vi "Process.vi"(8 "error in":errorcluster, 11 "system":refnum<class "system.lvclass">) -> (0 "error out":errorcluster, 3 "system out":refnum<class "system.lvclass">)   [LabVIEW 2016, in "system.lvclass"]
doc: "---------------------------------------------------------------\nJKI State Machine Objects™\nhttp://jki.net/state-machine-objects/\nCopyright (C) 2005-2015, JKI <info@jki.net>\nALL RIGHTS RESERVED"
uses:
  system.lvclass
  <vilib>/JKI/JKI SMO/SMO/SMO.lvclass
  <vilib>/JKI/JKI SMO/SMO/Typedefs/Parent Call--Enum.ctl
  instrument/instrument.lvclass
  DAQ_Manager/DAQ_Manager.lvclass
  DSP/DSP.lvclass
  C:/user/patrick/hg/levy_inst_lockin.SMO/lvsrc/SMOs/instrument/instrument.lvclass
  C:/Program Files (x86)/National Instruments/LabVIEW 2016/vi.lib/JKI/JKI SMO/SMO/SMO.lvclass
  Generator/Generator.lvclass
  DAQmx.AO/Typedefs/DAQmx.AO_Config.ctl
  DAQmx.AO/DAQmx.AO.lvclass
  DAQ/Typedefs/DAQ_Config.ctl
  DAQ/DAQ.lvclass
  DAQ/Typedefs/DAQ_SamplingMode.ctl
  DAQ/Typedefs/DAQ_SamplingInfo.ctl
  DAQ/Typedefs/PrivateEvents--DAQ.AI.Channels.ctl
  DAQ/Typedefs/DAQ_Type.ctl
  DAQmx.AI/Typedefs/DAQmx.AI_Config.ctl
  DAQmx.AI/DAQmx.AI.lvclass
  DAQmx.AI/Typedefs/AI.Coupling-enum.ctl
  DAQmx.AI/Typedefs/AI.Terminal-enum.ctl
  DAQmx.AO/Typedefs/AO.Terminal-enum.ctl
  DSP/Typedefs/LP_Config.ctl
  DSP.lockin/Typedefs/Lockin_Config.ctl
  DSP.lockin/DSP_lockin.lvclass
  <vilib>/Analysis/4window.llb/windowTd.ctl
  <vilib>/Analysis/NI_AALPro.lvlib
  <vilib>/measure/maspectr.llb/Power Spectrum and PSD Export Mode.ctl
  <vilib>/measure/NI_MAPro.lvlib
  DSP/Typedefs/FFT_Config.ctl
  DSP/Typedefs/PrivateEvents--DSP.RunCalculation.ctl
panel:
  in  "Tab Control":enum32{"process FP", "DAQ", "AO", "DSP"}(tab)
  in  "Simulate?":bool
  out "str":string
  in  "show UI?":bool
  in  "DAQmx Physical Channels (AI)":tag="PXI1Slot2/ai0:1, PXI1Slot3/ai0:1, PXI1Slot4/ai0:1, PXI1Slot5/ai0:1, PXI1Slot6/ai0:1, PXI1Slot7/ai0:1"
  in  "DAQmx.AO.config":T1={"output terminal configuration"=-1} {"output terminal configuration" items=["Default"=-1, "RSE"=10083, "Differential"=10106, "Pseudodifferential"=12529]}
  in  "DAQmx Physical Channels (AO)":tag="PXI1Slot2/ao0:1, PXI1Slot3/ao0:1, PXI1Slot4/ao0:1, PXI1Slot5/ao0:1, PXI1Slot6/ao0:1, PXI1Slot7/ao0:1"
  in  "DAQ.Config (AO)":T3={"Channels"="", "DAQ_Type"=enum."AO", "minimum value"=-10.0, "maximum value"=10.0, "DAQ_SamplingInfo"={"Fs"=1000.0, "#s"=1000}, "DAQ_SamplingMode"=enum."Continuous"} {"maximum value" format="%0.2f"; "minimum value" format="%0.2f"}
  in  "DAQ.Config (AI)":T3={"Channels"="", "DAQ_Type"=enum."AI", "minimum value"=-10.0, "maximum value"=10.0, "DAQ_SamplingInfo"={"Fs"=1000.0, "#s"=1000}, "DAQ_SamplingMode"=enum."Continuous"} {"maximum value" format="%0.2f"; "minimum value" format="%0.2f"}
  in  "DAQmx.AI.config":T8={"AI.Coupling"=10045, "input terminal configuration "=-1} {"input terminal configuration" items=["default"=-1, "RSE"=10083, "NRSE"=10078, "Differential"=10106, "Pseudodifferential"=12529]; "AI.Coupling" items=["AC"=10045, "DC"=10050, "GND"=10066]}
  in  "runCalculation":T11={"runCalculation"={"adjust gain"=FALSE, "subtract offset"=FALSE, "60 Hz prefilter"=FALSE, "LP prefilter"=FALSE, "lockin"=FALSE, "FFT"=FALSE, "gain"=[], "offset"=[], "LP config"={"high cutoff freq [Hz]"=0.45}, "Lockin config"=[], "FFT config"={"averaging parameters"={"averaging mode"=enum."RMS averaging", "weighting mode"=enum."Exponential", "number of averages"=10}, "window"=1, "export mode"=0, "window parameter"=nan, "restart averaging (F)"=FALSE}}} {"runCalculation"."FFT config"."export mode" items=["Power Spectrum", "Power Spectral Density"]; "runCalculation"."FFT config"."window" items=["Rectangle"=0, "Hanning"=1, "Hamming"=2, "Blackman-Harris"=3, "Exact Blackman"=4, "Blackman"=5, "Flat Top"=6, "4 Term B-Harris "=7, "7 Term B-Harris"=8, "Low Sidelobe"=9, "Blackman Nuttall"=11, "Triangle"=30, "Bartlett-Hanning"=31, "Bohman"=32, "Parzen"=33, "Welch"=34, "Kaiser"=60, "Dolph-Chebyshev"=61, "Gaussian"=62]; "runCalculation"."FFT config"."averaging parameters"."number of averages" min=1; "runCalculation"."Lockin config"."TC (s)" format="%#_13g"}
  # "system process.vi"
  # "For instructions on how to use the JKI State Machine Objects, examples and video tutorials, visit:\nhttp://jki.net/state-machine-objects/\n\nJKI State Machine Objects™\nhttp://jki.net/state-machine-objects/\nCopyright (C) 2005-2015, JKI <info@jki.net>\nALL RIGHTS RESERVED"
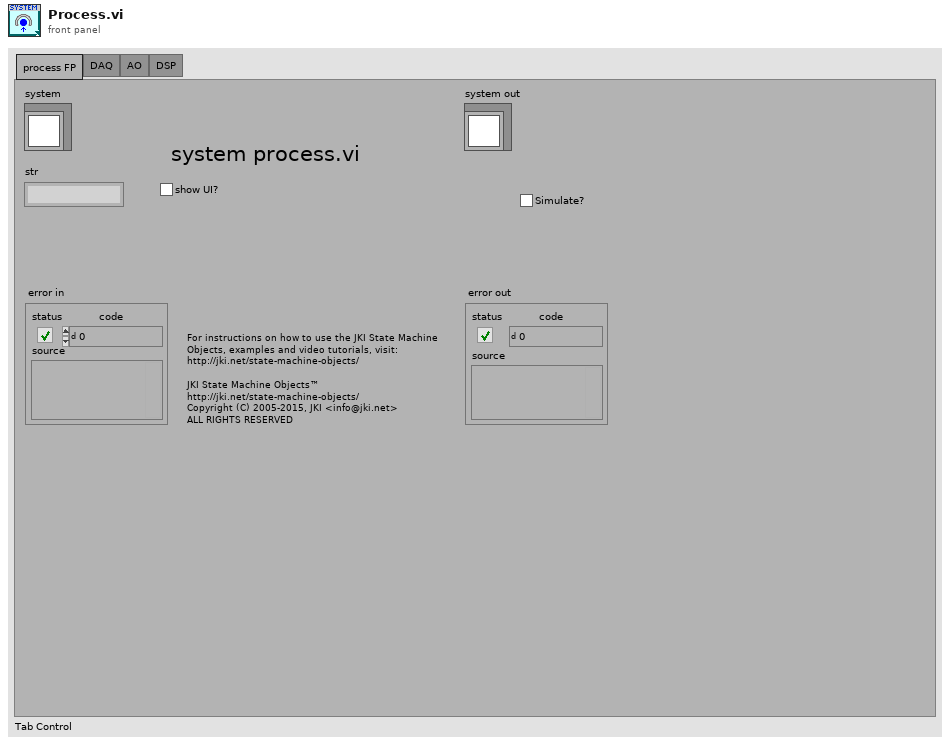
[diagram p1: front panel]
types:
  T1 = typedef "DAQmx.AO.lvclass/DAQmx.AO_Config.ctl" = cluster{"output terminal configuration":T2}
  T2 = typedef "DAQmx.AO.lvclass/AO.Terminal-enum.ctl" = i32
  T3 = typedef "DAQ.lvclass/DAQ_Config.ctl" = cluster{"Channels":T4, "DAQ_Type":T5, "minimum value":dbl, "maximum value":dbl, "DAQ_SamplingInfo":T6, "DAQ_SamplingMode":T7}
  T4 = typedef "DAQ.lvclass/PrivateEvents--DAQ.AI.Channels.ctl" = string
  T5 = typedef "DAQ.lvclass/DAQ_Type.ctl" = enum16{"AI", "AO"}
  T6 = typedef "DAQ.lvclass/DAQ_SamplingInfo.ctl" = cluster{"Fs":dbl, "#s":i32}
  T7 = typedef "DAQ.lvclass/DAQ_SamplingMode.ctl" = enum16{"Continuous", "Finite"}
  T8 = typedef "DAQmx.AI.lvclass/DAQmx.AI_Config.ctl" = cluster{"AI.Coupling":T9, "input terminal configuration ":T10}
  T9 = typedef "DAQmx.AI.lvclass/AI.Coupling-enum.ctl" = i32
  T10 = typedef "DAQmx.AI.lvclass/AI.Terminal-enum.ctl" = i32
  T11 = typedef "DSP.lvclass/PrivateEvents--DSP.RunCalculation.ctl" = cluster{"runCalculation":cluster{"adjust gain":bool, "subtract offset":bool, "60 Hz prefilter":bool, "LP prefilter":bool, "lockin":bool, "FFT":bool, "gain":dbl[], "offset":dbl[], "LP config":T12, "Lockin config":T13, "FFT config":T14}}
  T12 = typedef "DSP.lvclass/LP_Config.ctl" = cluster{"high cutoff freq [Hz]":dbl}
  T13 = typedef "DSP_lockin.lvclass/Lockin_Config.ctl" = cluster{" f (Hz)":dbl, "phi (deg)":dbl, "TC (s)":dbl, "order":i32}[]
  T14 = typedef "DSP.lvclass/FFT_Config.ctl" = cluster{"averaging parameters":cluster{"averaging mode":enum16{"No averaging", "Vector averaging", "RMS averaging", "Peak hold"}, "weighting mode":enum16{"Linear", "Exponential"}, "number of averages":u32}, "window":T15, "export mode":T16, "window parameter":dbl, "restart averaging (F)":bool}
  T15 = typedef "NI_AALPro.lvlib/windowTd.ctl" = u32
  T16 = typedef "NI_MAPro.lvlib/Power Spectrum and PSD Export Mode.ctl" = u16
  T17 = typedef "SMO.lvclass/Parent Call--Enum.ctl" = enum16{"Allows parent to run", "Does not request parent to run"}
  T18 = enum32{"invalid app kind", "Development System", "Run Time System", "Student Edition", "Embedded LabVIEW", "Evaluation", "Custom"}
  T19 = enum32{"Invalid", "Standard", "Closed", "Hidden", "Minimized", "Maximized"}
  T20 = enum32{"Bad", "Idle", "Run top level", "Running"}
  T21 = typedef "DAQ_Manager.lvclass/PublicEvents--DAQ_Manager.getWaveform.ctl" = waveform(dbl)[]
  T22 = cluster{"Core":cluster{"Current VI Reference":refnum<vi>, "Close Panel on Exit?":bool, "error":errorcluster}, "Self Reference":refnum<class "system.lvclass">, "Your string data":string, "to":i32, "AI Array":waveform(dbl)[], "AO Array":waveform(dbl)[], "DAQ_Manager":refnum<class "DAQ_Manager.lvclass">, "DSP":refnum<class "DSP.lvclass">, "Generator":refnum<class "Generator.lvclass">, "Scope":refnum<class "Scope.lvclass">}
  T23 = typedef "Generator.lvclass/PublicEvents--Generator.getGeneratorWaveforms.ctl" = waveform(dbl)[]
  T24 = cluster{"Current VI Reference":refnum<vi>, "Close Panel on Exit?":bool, "error":errorcluster}
  T25 = typedef "SMO.lvclass/Protected Events.ctl" = cluster{"StopProcesses":refnum<user-event>, "AbortProcesses":refnum<user-event>, "Config Changed":refnum<user-event>, "Dependency":refnum<user-event>}
  T26 = typedef "system.lvclass/PrivateEvents--Cluster.ctl" = cluster{"output_config":refnum<user-event>, "lockin_config":refnum<user-event>, "lockin_REF_waveform":refnum<user-event>}
  T27 = cluster{"SMO Protected Events":T25, "Private Events":T26}
  T28 = typedef "SMO.lvclass/Public Events.ctl" = cluster{"Error":refnum<user-event>, "State":refnum<user-event>, "Reserve State":refnum<user-event>}
  T29 = typedef "DAQ_Manager.lvclass/PublicEvents--Cluster.ctl" = cluster{"getWaveform":refnum<user-event>}
  T30 = cluster{"Public Events":T28, "Public Events":T29}
  T31 = typedef "DSP.lvclass/PublicEvents--Cluster.ctl" = cluster{"getWaveforms":refnum<user-event>, "getLockin":refnum<user-event>, "getPowerSpectrum":refnum<user-event>}
  T32 = cluster{"Public Events":T28, "Public Events":T31}
  T33 = typedef "Generator.lvclass/PublicEvents--Cluster.ctl" = cluster{"getGeneratorWaveforms":refnum<user-event>}
  T34 = cluster{"Public Events":T28, "Public Events":T33}
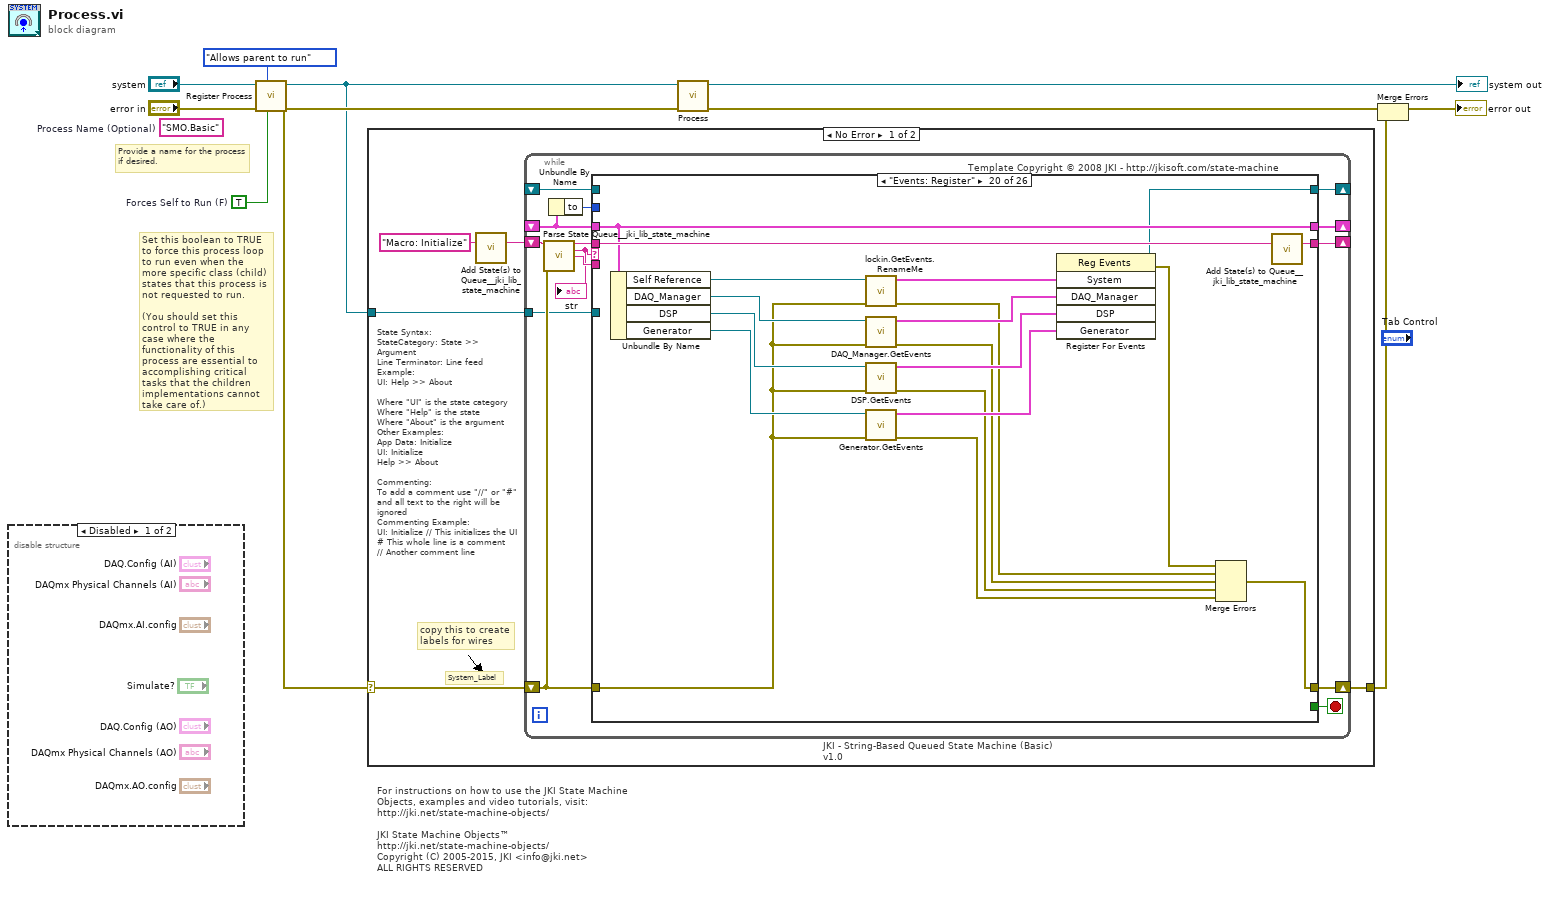
[diagram p0: block diagram]
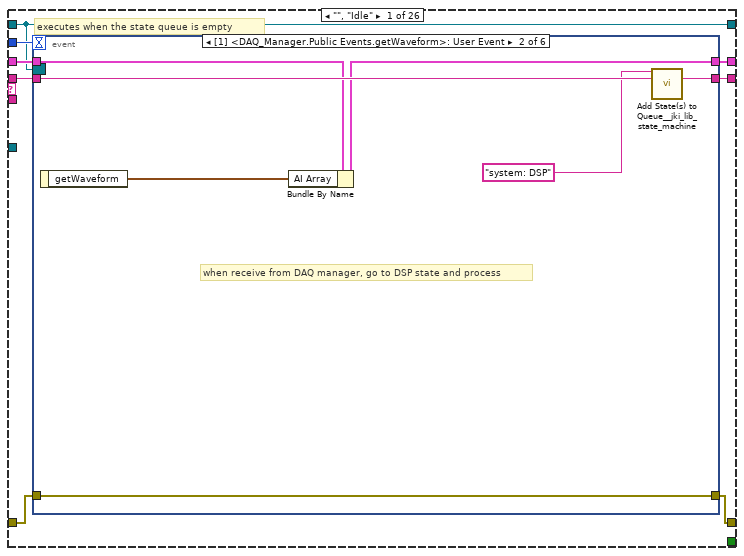
[diagram p3: hidden frame]
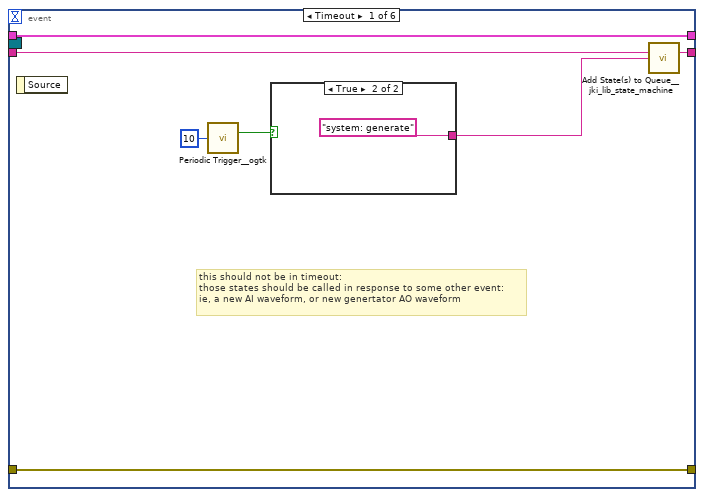
[diagram p4: hidden frame]
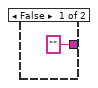
[diagram p5: hidden frame]
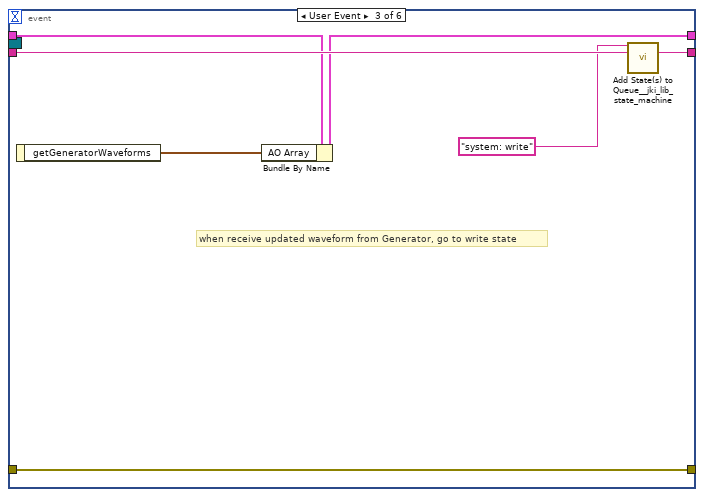
[diagram p6: hidden frame]
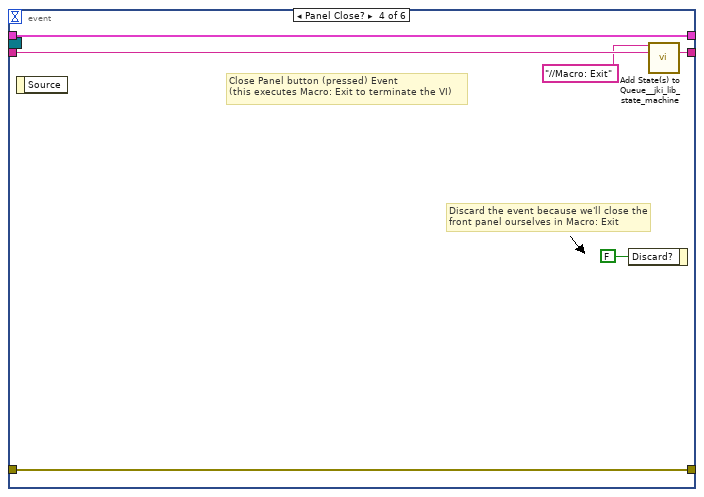
[diagram p7: hidden frame]
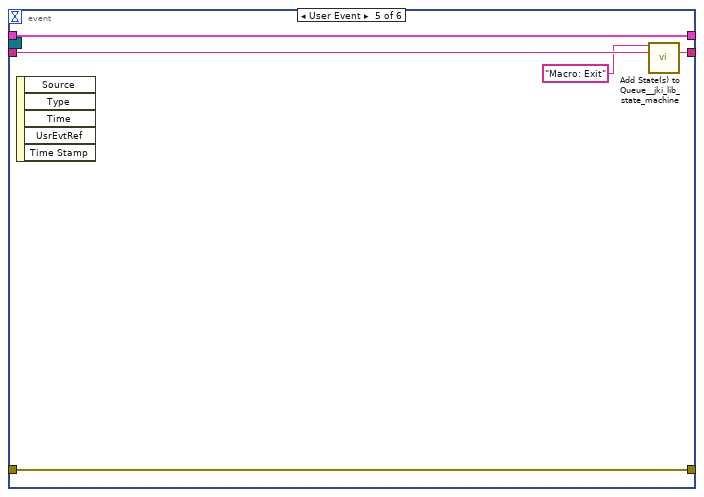
[diagram p8: hidden frame]
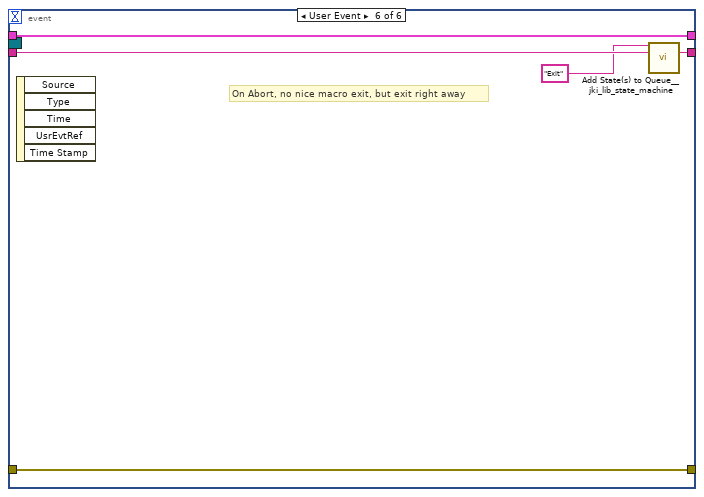
[diagram p9: hidden frame]
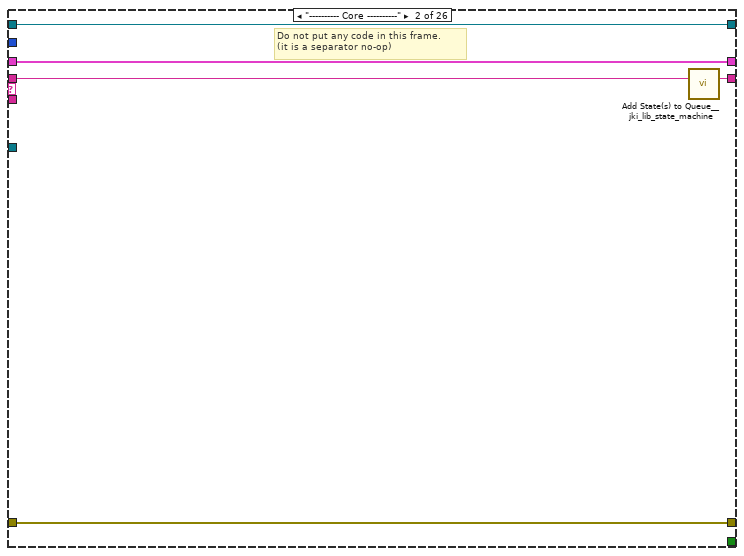
[diagram p10: hidden frame]
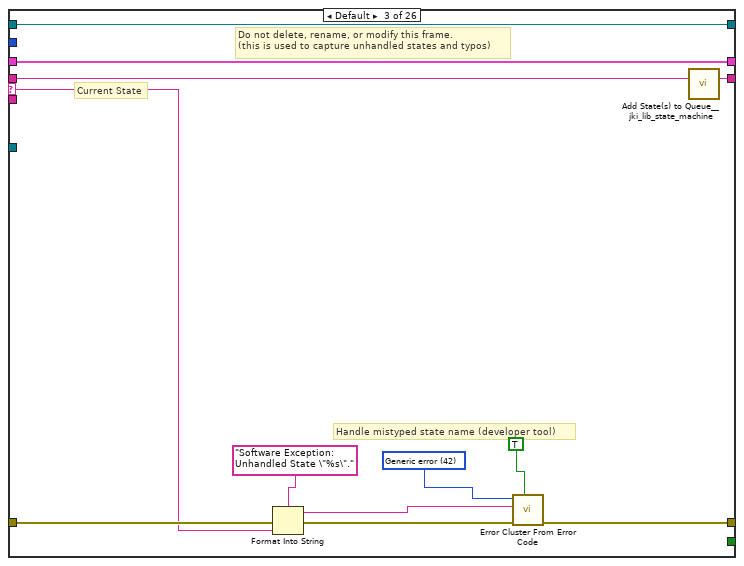
[diagram p11: hidden frame]
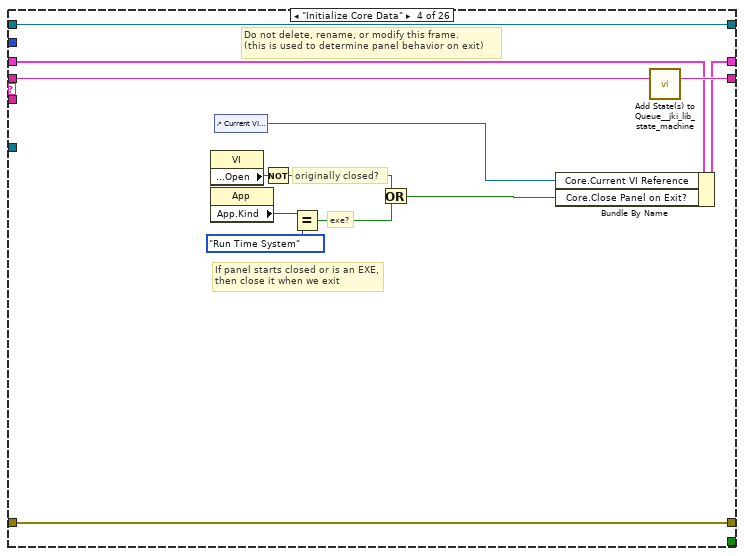
[diagram p12: hidden frame]
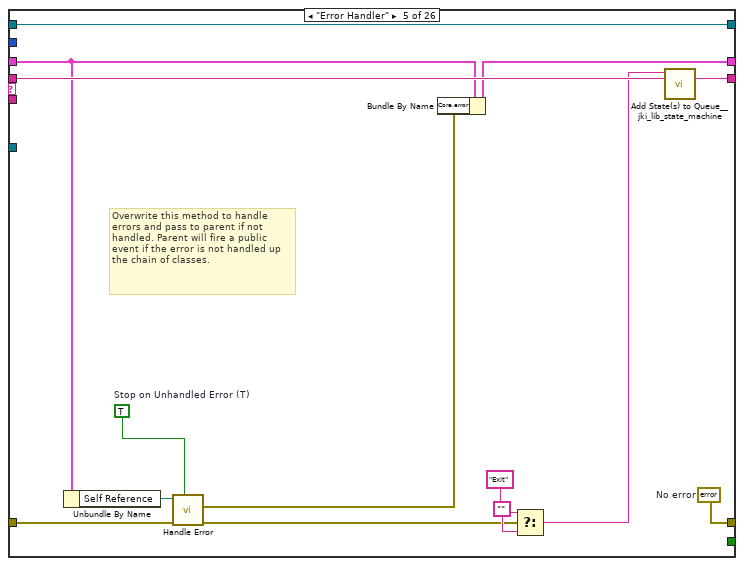
[diagram p13: hidden frame]
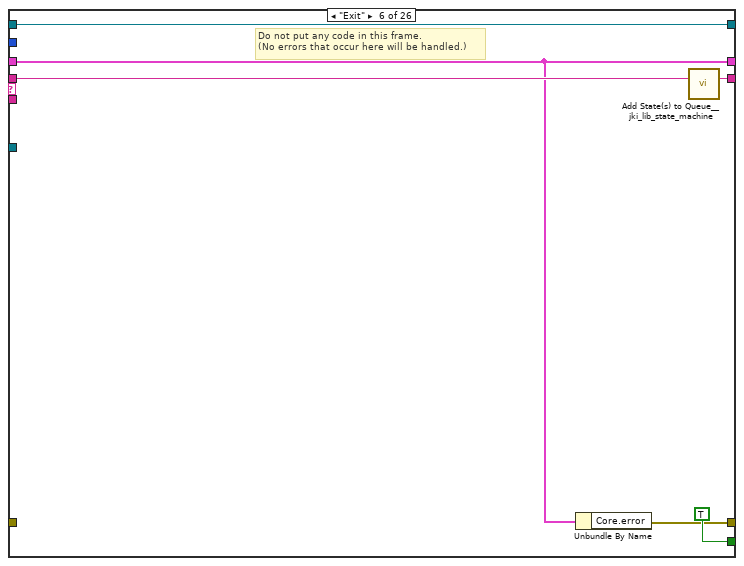
[diagram p14: hidden frame]
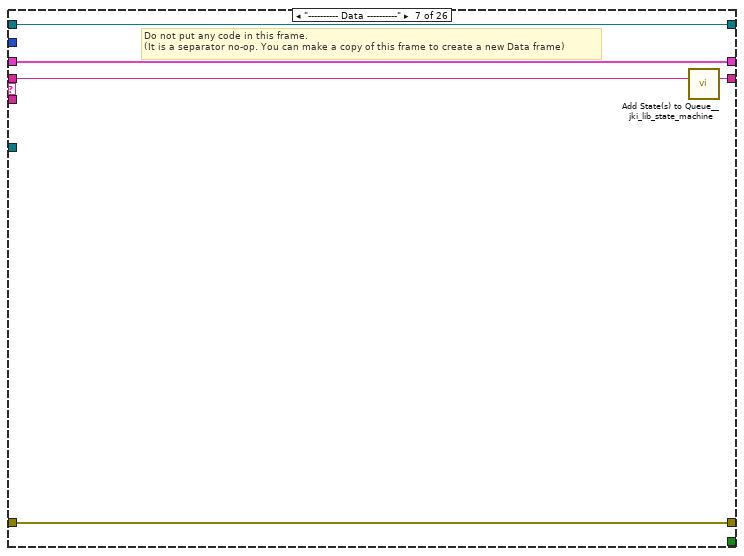
[diagram p15: hidden frame]
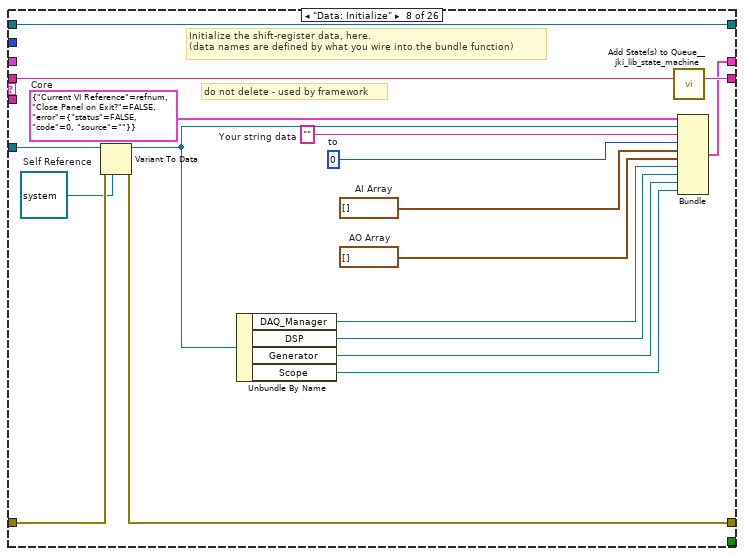
[diagram p16: hidden frame]
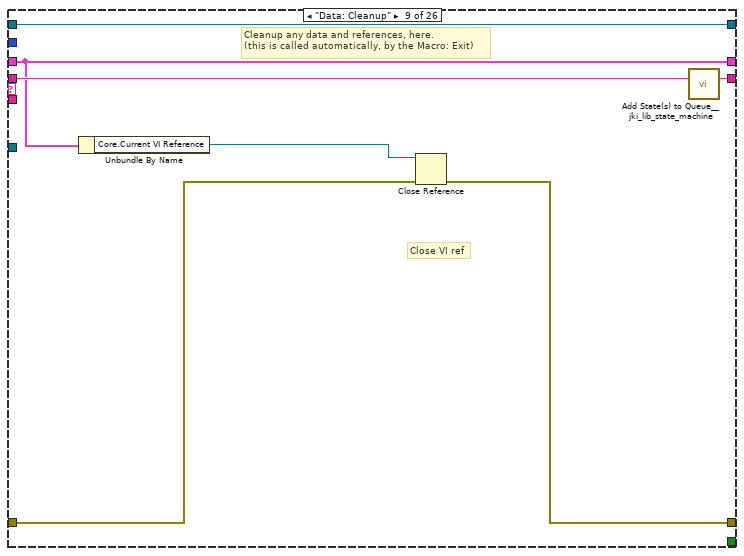
[diagram p17: hidden frame]
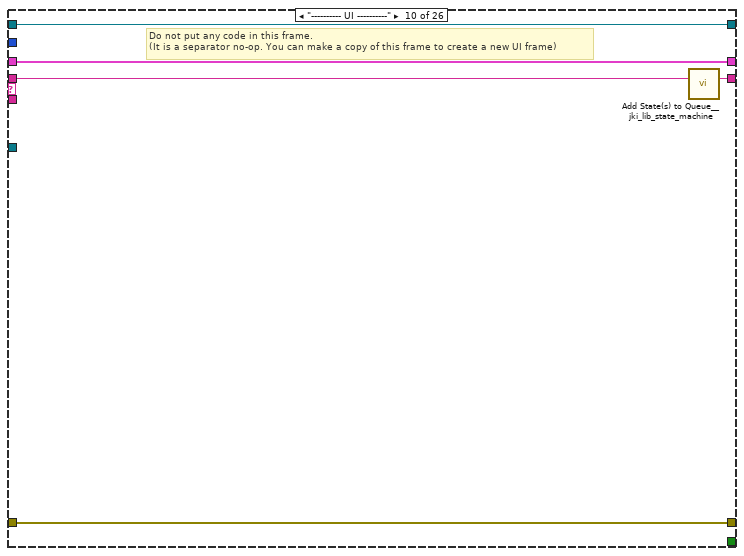
[diagram p18: hidden frame]
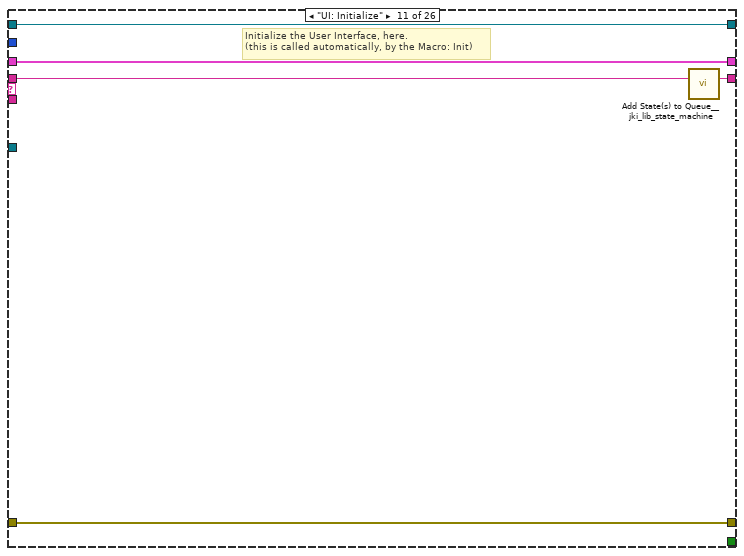
[diagram p19: hidden frame]
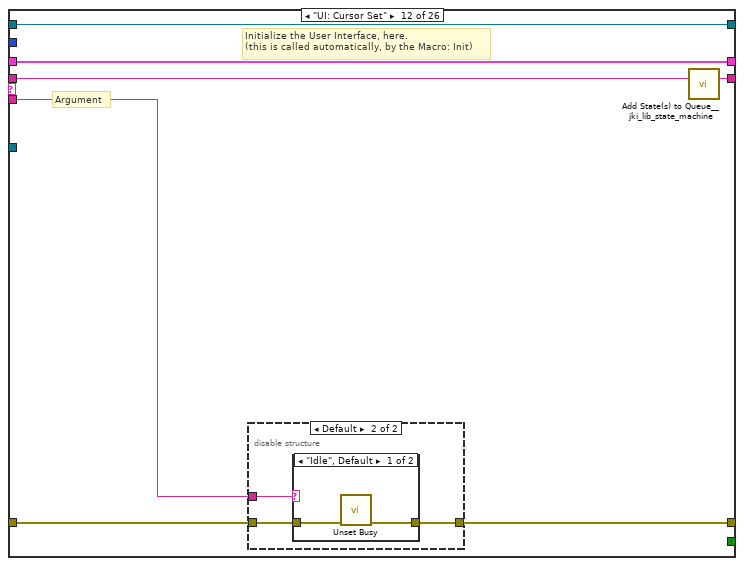
[diagram p20: hidden frame]
diagram:
  w1 = TRUE  # Forces Self to Run (F)
  (unwired) "SMO.Basic"  # Process Name (Optional)
  # "Provide a name for the process\nif desired."
  # "Set this boolean to TRUE to force this process loop to run even when the more specific class (child) states that this process is not requested to run.\n\n(You should set this control to TRUE in any case where the functionality of this process are essential to accomplishing critical tasks that the children implementations cannot take care of.)"
  # "For instructions on how to use the JKI State Machine Objects, examples and video tutorials, visit:\nhttp://jki.net/state-machine-objects/\n\nJKI State Machine Objects™\nhttp://jki.net/state-machine-objects/\nCopyright (C) 2005-2015, JKI <info@jki.net>\nALL RIGHTS RESERVED"
  n1 = disable-structure shown="Disabled" {
    frame Disabled {
    }
    frame Enabled {
    }
  }
  n2 = call <vilib>:"Register Process.vi"("Forces Self to Run (F)"=w1, "Parent Call"=Parent_Call--Enum."Allows parent to run", "error in (no error)"="error in", "SMO"="system") -> ("error out"=w7:errorcluster, "SMO out"=w6:refnum<class "system.lvclass">)  [unwired: 6 in]
  n3 = case shown="No Error" w7 {
    selector: w7 -> [w12 w346]
    tunnel: w6 -> [w13 _]
    tunnel: [w11 w346] -> w3
    frame No Error {
      # "State Syntax:\nStateCategory: State >> Argument\nLine Terminator: Line feed\nExample:\nUI: Help >> About\n\nWhere \"UI\" is the state category\nWhere \"Help\" is the state\nWhere \"About\" is the argument\nOther Examples:\nApp Data: Initialize\nUI: Initialize\nHelp >> About\n\nCommenting:\nTo add a comment use \"//\" or \"#\" and all text to the right will be ignored\nCommenting Example:\nUI: Initialize // This initializes the UI\n# This whole line is a comment\n// Another comment line"
      # "copy this to create labels for wires"
      # "System_Label"
      n4 = call <vilib>:"Add State(s) to Queue__jki_lib_state_machine.vi"("State(s) in (\"\")"="Macro: Initialize") -> ("States Out"=w15:string)  [unwired: 14 in]
      n5 = while "JKI - String-Based Queued State Machine (Basic) v1.0" {
        shift-right: [w23] -> _
        shift-left: _ -> [w17]
        shift-right: [w26] -> w11
        shift-left: w12 -> [w22]
        shift-right: [w25] -> _
        shift-left: w15 -> [w27]
        tunnel: w13 -> [w21]
        shift-right: [w20] -> _
        shift-left: _ -> [w19]
        stop <- w24 stop-if-true
        # "Template Copyright © 2008 JKI - http://jkisoft.com/state-machine"
        n6 = call <vilib>:"Parse State Queue__jki_lib_state_machine.vi"("State Queue"=w27, "Error In (no error)"=w22) -> ("Remaining States"=w29:string, "Current State"=w18:string, "Arguments"=w28:string)  [unwired: 11 in]
        "str" <- w18
        n7 = Unbundle By Name(w17) -> ("to"=w16:i32)
        n8 = case shown="\"Events: Register\"" w18 {
          selector: w18 -> [_ _ w83 _ _ _ _ _ _ _ _ _ _ _ _ _ _ _ _ _ _ _ _ _ _ _]
          tunnel: w29 -> [w37 w81 w87 w106 w120 w126 w131 w149 w156 w161 w166 w173 w189 w221 w241 w255 w260 w271 w276 w295 w301 w306 w313 w325 w335 w345]
          tunnel: w28 -> [_ _ _ _ _ _ _ _ _ _ _ w167 w183 _ _ _ _ _ _ _ _ _ _ _ _ _]
          tunnel: w17 -> [w35 w78 w85 w97 w114 w122 w128 _ w152 w158 w164 w171 w185 w218 w237 w246 w257 w268 w273 w293 w299 w304 w310 w321 w331 w342]
          tunnel: [w34 w79 w89 w103 w115 w121 w129 w144 w153 w159 w163 w168 w186 w219 w239 w253 w258 w262 w274 w278 w297 w302 w307 w317 w330 w341] -> w26
          tunnel: w22 -> [w33 w79 w88 w103 w116 _ w129 w145 w151 w159 w163 w169 w187 w219 w239 w253 w258 w263 w274 w284 w297 w302 w307 w319 w330 w337]
          tunnel: [w36 w80 w86 w105 w119 w125 w130 w148 w155 w160 w165 w172 w188 w220 w240 w254 w259 w270 w275 w294 w300 w305 w312 w324 w334 w344] -> w25
          tunnel: [_ _ _ _ _ TRUE _ _ _ _ _ _ _ _ _ _ _ _ _ _ _ _ _ _ _ _] -> w24
          tunnel: [w32 w78 w85 w104 w113 w122 w128 w147 w152 w158 w164 w171 w185 w218 w237 w246 w257 w268 w273 w293 w299 w304 w309 w321 w331 w342] -> w23
          tunnel: w16 -> [w31 _ _ _ _ _ _ _ _ _ _ _ _ _ _ _ _ _ _ _ _ _ _ _ _ _]
          tunnel: w21 -> [_ _ _ _ _ _ _ w142 _ _ _ _ _ _ _ _ _ _ _ _ _ _ _ _ _ _]
          tunnel: [w30 w77 w82 w94 w118 w123 w127 w141 w154 w157 w162 w170 w182 w217 w238 w247 w256 w269 w272 w287 w298 w303 w311 w323 w333 w343] -> w20
          tunnel: w19 -> [w30 w77 w82 w94 w118 w123 w127 w141 w154 w157 w162 w170 w182 w217 w238 w247 w256 w269 w272 _ w298 w303 w311 w323 w333 w343]
          frame "", "Idle" {
            # "executes when the state queue is empty"
            n9 = event shown="[1] <DAQ_Manager.Public Events.getWaveform>: User Event" {
              selector: w30 -> [_ _ _ _ _ _]
              dyn-events: _ -> [_ _ _ _ _ _]
              timeout: w31 -> [_ _ _ _ _ _]
              tunnel: w37 -> [w44 w52 w59 w66 w71 w76]
              tunnel: [w43 w53 w60 w65 w70 w75] -> w36
              tunnel: w35 -> [w42 w50 w57 w63 w68 w73]
              tunnel: [w41 w51 w58 w64 w69 w74] -> w34
              tunnel: w33 -> [w41 w51 w58 w64 w69 w74]
              tunnel: [w42 w49 w56 w63 w68 w73] -> w32
              event Timeout {
                # "this should not be in timeout:\nthose states should be called in response to some other event:\nie, a new AI waveform, or new genertator AO waveform"
                n10 = event-data() -> ()  [unwired: 1 in, 1 out]
                n11 = call <userlib>:"Periodic Trigger__ogtk.vi"("time (ms)"=u32 10) -> ("Triggered"=w38:bool)  [unwired: 12 in, 2 out]
                n12 = case shown="True" w38 {
                  tunnel: ["" ("State(s) in Front (\"\")") "system: generate" ("State(s) in Front (\"\")")] -> w40
                  frame False {
                  }
                  frame True {
                  }
                }
                n13 = call <vilib>:"Add State(s) to Queue__jki_lib_state_machine.vi"("State(s) in (\"\")"=w44, "State(s) at Back (\"\")"=w40) -> ("States Out"=w43:string)  [unwired: 13 in]
              }
              event User Event {
                # "when receive from DAQ manager, go to DSP state and process"
                n14 = event-data() -> ("getWaveform"=w48:T21)  [unwired: 1 in]
                n15 = Bundle By Name(cluster=w50, "AI Array"=w48) -> (w49:T22)
                n16 = call <vilib>:"Add State(s) to Queue__jki_lib_state_machine.vi"("State(s) in Front (\"\")"="system: DSP" ("State(s) in Front (\"\")"), "State(s) in (\"\")"=w52) -> ("States Out"=w53:string)  [unwired: 13 in]
              }
              event User Event {
                # "when receive updated waveform from Generator, go to write state"
                n17 = event-data() -> ("getGeneratorWaveforms"=w55:T23)  [unwired: 1 in]
                n18 = Bundle By Name(cluster=w57, "AO Array"=w55) -> (w56:T22)
                n19 = call <vilib>:"Add State(s) to Queue__jki_lib_state_machine.vi"("State(s) in Front (\"\")"="system: write" ("State(s) in Front (\"\")"), "State(s) in (\"\")"=w59) -> ("States Out"=w60:string)  [unwired: 13 in]
              }
              event Panel Close? {
                # "Discard the event because we'll close the front panel ourselves in Macro: Exit"
                # "Close Panel button (pressed) Event\n(this executes Macro: Exit to terminate the VI)"
                n20 = event-data() -> ()  [unwired: 1 in, 1 out]
                n21 = event-data("Discard?"=FALSE) -> ()  [unwired: 1 in, 1 out]
                n22 = call <vilib>:"Add State(s) to Queue__jki_lib_state_machine.vi"("State(s) in Front (\"\")"="//Macro: Exit", "State(s) in (\"\")"=w66) -> ("States Out"=w65:string)  [unwired: 13 in]
              }
              event User Event {
                n23 = event-data() -> ()  [unwired: 1 in, 5 out]
                n24 = call <vilib>:"Add State(s) to Queue__jki_lib_state_machine.vi"("State(s) in Front (\"\")"="Macro: Exit", "State(s) in (\"\")"=w71) -> ("States Out"=w70:string)  [unwired: 13 in]
              }
              event User Event {
                # "On Abort, no nice macro exit, but exit right away"
                n25 = event-data() -> ()  [unwired: 1 in, 5 out]
                n26 = call <vilib>:"Add State(s) to Queue__jki_lib_state_machine.vi"("State(s) in Front (\"\")"="Exit", "State(s) in (\"\")"=w76) -> ("States Out"=w75:string)  [unwired: 13 in]
              }
            }
          }
          frame "---------- Core ----------" {
            # "Do not put any code in this frame.\n(it is a separator no-op)"
            n27 = call <vilib>:"Add State(s) to Queue__jki_lib_state_machine.vi"("State(s) in (\"\")"=w81) -> ("States Out"=w80:string)  [unwired: 14 in]
          }
          frame Default {
            w92 = 42 items=["No error", "Argument error", "Memory is full", "Out of zone", "End of file", "File already open", "Generic file I/O error", "File not found", "File permission error", "Disk is full", "Duplicate path", "Too many files open", "System feature not enabled", "Resource file not found", "Cannot add resource", "Resource not found", "Image not found", "Image memory error", "Pen does not exist", "Config type invalid", "Config token not found", "Config parse error", "Config memory error", "Bad external code format", "Bad external code offset", "External code not present", "Null window", "Destroy window error", "Null menu", "Print aborted", "Bad print record", "Print driver error", "Windows error during printing", "Memory error during printing", "Print dialog error", "Generic print error", "Invalid device refnum", "Device not found", "Device parameter error", "Device unit error", "Cannot open device", "Device call aborted", "Generic error", "Cancelled by user", "Object ID too low", "Object ID too high", "Object not in heap", "Unknown heap", "Unknown object (invalid DefProc)", "Unknown object (DefProc not in table)", "Message out of range", "Invalid (null) method", "Unknown message", "Manager call not supported", "Bad address", "Network operation in progress", "Network operation timed out", "Connection is busy", "Network attribute not supported", "Network error", "Address in use", "System out of memory", "Connection aborted", "Connection refused", "Not connected", "Already connected", "Connection closed", "Initialization error (interapplication manager)", "Bad occurrence", "Wait on unbound occurrence handler", "Occurrence queue overflow", "Datalog type conflict", "Unused", "Unrecognized type (interapplication manager)", "Memory corrupt", "Failed to make temporary DLL", "Old CIN version", "Drag socket not found", "Failed to load drop-object", "Failed to register OLE object", "Failed to release OLE object", "Format specifier type mismatch", "Unknown format specifier", "Too few format specifiers", "Too many format specifiers", "Scan failed", "Newer CIN version", "Error converting to variant", "Runtime menu error", "Password tampered", "Variant attribute not found", "Incompatible variant data type", "Event data is not available", "Event Store is not present", "Occurrence is not found", "Event Queue is not created", "Event info is not available", "Refnum passed is NULL", "Error retrieving Class GUID", "Error retrieving CoClass GUID", "Error retrieving TypeLib GUID.", "Bad built application magic bytes.", "Specific driver is different from the specific driver associated with the Logical Name.", "There is no session opened to the class driver.", "Max Error", "MAX - Error with config objects", "MAX - Error loading configuration", "MAX - Group not supported"]
            # "Current State"
            # "Do not delete, rename, or modify this frame.\n(this is used to capture unhandled states and typos)"
            # "Handle mistyped state name (developer tool)"
            n28 = Format Into String(format string="Software Exception: Unhandled State \"%s\"." ("message"), error in=w88, w83) -> (resulting string=w91:string, error out=w90:errorcluster)  [unwired: 1 in]
            n29 = call <vilib>:"Error Cluster From Error Code.vi"("show call chain? (False)"=TRUE, "error in (no error)"=w90, "error message (\"\")"=w91, "error code (0)"=w92) -> ("error out"=w89:errorcluster)  [unwired: 5 in]
            n30 = call <vilib>:"Add State(s) to Queue__jki_lib_state_machine.vi"("State(s) in (\"\")"=w87) -> ("States Out"=w86:string)  [unwired: 14 in]
          }
          frame "Initialize Core Data" {
            # "Do not delete, rename, or modify this frame.\n(this is used to determine panel behavior on exit)"
            # "originally closed?"
            # "exe?"
            # "If panel starts closed or is an EXE, then close it when we exit"
            n31 = property class="VI"() -> ("Front Panel.Open"=w102:bool)  [unwired: 2 in, 2 out]
            n32 = property class="App"() -> ("App.Kind"=w101:T18)  [unwired: 2 in, 2 out]
            n33 = control-ref of="Current VI Reference"() -> (w95:refnum<vi>)
            n34 = Not(x=w102) -> (.not. x?=w99:bool)
            n35 = Equal?(x=w101, y=T18."Run Time System" ("Application:Kind")) -> (x = y?=w98:bool)
            n36 = Or(x=w99, y=w98) -> (x .or. y?=w96:bool)
            n37 = Bundle By Name(cluster=w97, "Core.Current VI Reference"=w95, "Core.Close Panel on Exit?"=w96) -> (w104:T22)
            n38 = call <vilib>:"Add State(s) to Queue__jki_lib_state_machine.vi"("State(s) in (\"\")"=w106) -> ("States Out"=w105:string)  [unwired: 14 in]
          }
          frame "Error Handler" {
            w107 = TRUE  # Stop on Unhandled Error (T)
            w115 = errorcluster {"status"=FALSE, "code"=0, "source"=""}  # No error
            # "Overwrite this method to handle errors and pass to parent if not handled. Parent will fire a public event if the error is not handled up the chain of classes."
            n39 = Unbundle By Name(w114) -> ("Self Reference"=w117:refnum<class "system.lvclass">)
            n40 = call-dynamic "Handle Error.vi"("Stop on Unhandled Error (T)"=w107, "error in"=w116, "SMO"=w117) -> ("handling error"=w108:errorcluster, "Unhandled error"=w111:errorcluster)  [unwired: 6 in, 1 out]
            n41 = Bundle By Name(cluster=w114, "Core.error"=w111) -> (w113:T22)
            n42 = Select(t="Exit", s=w108, f="") -> (s? t:f=w112:string)
            n43 = call <vilib>:"Add State(s) to Queue__jki_lib_state_machine.vi"("State(s) in Front (\"\")"=w112, "State(s) in (\"\")"=w120) -> ("States Out"=w119:string)  [unwired: 13 in]
          }
          frame "Exit" {
            # "Do not put any code in this frame.\n(No errors that occur here will be handled.)"
            n44 = Unbundle By Name(w122) -> ("Core.error"=w121:errorcluster)
            n45 = call <vilib>:"Add State(s) to Queue__jki_lib_state_machine.vi"("State(s) in (\"\")"=w126) -> ("States Out"=w125:string)  [unwired: 14 in]
          }
          frame "---------- Data ----------" {
            # "Do not put any code in this frame.\n(It is a separator no-op. You can make a copy of this frame to create a new Data frame)"
            n46 = call <vilib>:"Add State(s) to Queue__jki_lib_state_machine.vi"("State(s) in (\"\")"=w131) -> ("States Out"=w130:string)  [unwired: 14 in]
          }
          frame "Data: Initialize" {
            w137 = waveform(dbl)[] []  # AO Array
            w138 = waveform(dbl)[] []  # AI Array
            w139 = 0  # to
            w140 = T24 {"Current VI Reference"=refnum, "Close Panel on Exit?"=FALSE, "error"={"status"=FALSE, "code"=0, "source"=""}}  # Core
            w143 = refnum<class "system.lvclass"> refnum  # Self Reference
            w146 = ""  # Your string data
            # "do not delete - used by framework"
            # "Initialize the shift-register data, here.\n(data names are defined by what you wire into the bundle function)"
            n47 = Variant To Data(error in=w145, type=w143, Variant=w142) -> (data=w136:refnum<class "system.lvclass">, error out=w144:errorcluster)
            n48 = Unbundle By Name(w136) -> ("DAQ_Manager"=w135:refnum<class "DAQ_Manager.lvclass">, "DSP"=w134:refnum<class "DSP.lvclass">, "Generator"=w133:refnum<class "Generator.lvclass">, "Scope"=w132:refnum<class "Scope.lvclass">)
            n49 = call <vilib>:"Add State(s) to Queue__jki_lib_state_machine.vi"("State(s) in (\"\")"=w149) -> ("States Out"=w148:string)  [unwired: 14 in]
            n50 = Bundle("Core"=w140, "Self Reference"=w136, "Your string data"=w146, "to"=w139, "AI Array"=w138, "AO Array"=w137, "DAQ_Manager"=w135, "DSP"=w134, "Generator"=w133, "Scope"=w132) -> (w147:T22)  [unwired: 1 in]
          }
          frame "Data: Cleanup" {
            # "Close VI ref"
            # "Cleanup any data and references, here.\n(this is called automatically, by the Macro: Exit)"
            n51 = Unbundle By Name(w152) -> ("Core.Current VI Reference"=w150:refnum<vi>)
            n52 = Close Reference(reference=w150, error in (no error)=w151) -> (error out=w153:errorcluster)
            n53 = call <vilib>:"Add State(s) to Queue__jki_lib_state_machine.vi"("State(s) in (\"\")"=w156) -> ("States Out"=w155:string)  [unwired: 14 in]
          }
          frame "---------- UI ----------" {
            # "Do not put any code in this frame.\n(It is a separator no-op. You can make a copy of this frame to create a new UI frame)"
            n54 = call <vilib>:"Add State(s) to Queue__jki_lib_state_machine.vi"("State(s) in (\"\")"=w161) -> ("States Out"=w160:string)  [unwired: 14 in]
          }
          frame "UI: Initialize" {
            # "Initialize the User Interface, here.\n(this is called automatically, by the Macro: Init)"
            n55 = call <vilib>:"Add State(s) to Queue__jki_lib_state_machine.vi"("State(s) in (\"\")"=w166) -> ("States Out"=w165:string)  [unwired: 14 in]
          }
          frame "UI: Cursor Set" {
            # "Argument"
            # "Initialize the User Interface, here.\n(this is called automatically, by the Macro: Init)"
            n56 = disable-structure shown="Default" {
              disable-tunnel: w169 -> [w174 w177]
              disable-tunnel: [w174 w176] -> w168
              disable-tunnel: w167 -> [_ w175]
              frame condition #0 {
              }
              frame condition #1 (active) {
                n57 = case shown="\"Idle\", Default" w175 {
                  tunnel: w177 -> [w179 w181]
                  tunnel: [w178 w180] -> w176
                  frame "Idle", Default {
                    n58 = call <vilib>:"Unset Busy.vi"("error in (no error)"=w179) -> ("error out"=w178:errorcluster)  [unwired: 10 in]
                  }
                  frame "Busy" {
                    n59 = call <vilib>:"Set Busy.vi"("error in (no error)"=w181) -> ("error out"=w180:errorcluster)  [unwired: 9 in, 1 out]
                  }
                }
              }
            }
            n60 = call <vilib>:"Add State(s) to Queue__jki_lib_state_machine.vi"("State(s) in (\"\")"=w173) -> ("States Out"=w172:string)  [unwired: 14 in]
          }
          frame "UI: Front Panel State" {
            # "Argument"
            # "Set Front Panel Open or Closed\n(Usage: \"UI: Front Panel State >> Open|Close\")"
            n61 = Unbundle By Name(w185) -> ("Core.Current VI Reference"=w184:refnum<vi>)
            n62 = disable-structure shown="Default" {
              disable-tunnel: w187 -> [w193 w216]
              disable-tunnel: [w192 w216] -> w186
              disable-tunnel: w184 -> [w191 _]
              disable-tunnel: w183 -> [w190 _]
              frame condition #0 (active) {
                n63 = case shown="\"Close\"" w190 {
                  tunnel: w193 -> [w197 w210]
                  tunnel: [w199 w211] -> w192
                  tunnel: w191 -> [w198 w208]
                  frame "Open", Default {
                    n64 = property class="VI"(reference=w198, error in=w197) -> (reference out=w195:refnum<vi>, error out=w196:errorcluster, "FP.State"=w194:T19)
                    n65 = case shown="\"Closed\"" w194 {
                      tunnel: [w202 w205] -> w199
                      tunnel: w196 -> [w201 w205]
                      tunnel: w195 -> [w200 _]
                      frame "Closed" {
                        n66 = invoke class="VI" method="FP.Open"(reference=w200, error in=w201, "Activate"=TRUE, "State"=T19."Standard") -> (error out=w202:errorcluster)  [unwired: 1 in, 4 out]
                      }
                      frame Default {
                      }
                    }
                  }
                  frame "Close" {
                    n67 = property class="VI"(reference=w208, error in=w210) -> (reference out=w207:refnum<vi>, error out=w209:errorcluster, "FP.State"=w206:T19)
                    n68 = case shown="Default" w206 {
                      tunnel: [w212 w215] -> w211
                      tunnel: w209 -> [w212 w214]
                      tunnel: w207 -> [_ w213]
                      frame "Invalid", "Closed" {
                      }
                      frame Default {
                        n69 = invoke class="VI" method="FP.Close"(reference=w213, error in=w214) -> (error out=w215:errorcluster)  [unwired: 1 in, 2 out]
                      }
                    }
                  }
                }
              }
              frame condition #1 {
              }
            }
            n70 = call <vilib>:"Add State(s) to Queue__jki_lib_state_machine.vi"("State(s) in (\"\")"=w189) -> ("States Out"=w188:string)  [unwired: 14 in]
          }
          frame "---------- Macro ----------" {
            # "Do not put any code in this frame.\n(It is a separator no-op. You can make a copy of this frame to create a new Macro frame)"
            n71 = call <vilib>:"Add State(s) to Queue__jki_lib_state_machine.vi"("State(s) in (\"\")"=w221) -> ("States Out"=w220:string)  [unwired: 14 in]
          }
          frame "Macro: Initialize" {
            w229 = "Process: Sync"
            # "Initialization Macro\n(This is called once, when the VI starts)"
            n72 = control-ref of="This VI"() -> (w231:refnum<vi>)
            n73 = property class="VI"(reference=w231) -> ("Exec.State"=w230:T20)  [unwired: 1 in, 2 out]
            n74 = Equal?(x=w230, y=T20."Run top level") -> (x = y?=w235:bool)
            n75 = Select(t="Open", s="show UI?", f="Close") -> (s? t:f=w224:string)
            n76 = Select(t=w229, s=w235, f="") -> ()  [unwired: 1 out]
            n77 = Concatenate Strings("UI: Front Panel State >> ", w224) -> (w223:string)
            n78 = call <vilib>:"Add State(s) to Queue__jki_lib_state_machine.vi"("State(s) in Front (\"\")"=w223) -> ("States Out"=w222:string)  [unwired: 14 in]
            n79 = call <vilib>:"Add State(s) to Queue__jki_lib_state_machine.vi"("State(s) in Front (\"\")"="Data: Initialize\nInitialize Core Data\nEvents: Register", "State(s) in (\"\")"=w229, "State(s) at Back (\"\")"=w222) -> ("States Out"=w232:string)  [unwired: 12 in]
            n80 = call <vilib>:"Add State(s) to Queue__jki_lib_state_machine.vi"("State(s) in Front (\"\")"=w232, "State(s) in (\"\")"=w241) -> ("States Out"=w240:string)  [unwired: 13 in]
          }
          frame "Macro: Exit" {
            # "Exit Macro\n(This is called once, when the VI exits)"
            n81 = Unbundle By Name(w246) -> ("Core.Close Panel on Exit?"=w252:bool)
            n82 = Select(t="UI: Front Panel State >> Close", s=w252, f="") -> (s? t:f=w249:string)
            n83 = call <vilib>:"Add State(s) to Queue__jki_lib_state_machine.vi"("State(s) in Front (\"\")"="Data: Cleanup\nEvents: Unregister", "State(s) in (\"\")"="Process: Sync", "State(s) at Back (\"\")"="Exit") -> ("States Out"=w243:string)  [unwired: 12 in]
            n84 = call <vilib>:"Add State(s) to Queue__jki_lib_state_machine.vi"("State(s) in (\"\")"=w249, "State(s) at Back (\"\")"=w243) -> ("States Out"=w248:string)  [unwired: 13 in]
            n85 = call <vilib>:"Add State(s) to Queue__jki_lib_state_machine.vi"("State(s) in Front (\"\")"=w248, "State(s) in (\"\")"=w255) -> ("States Out"=w254:string)  [unwired: 13 in]
          }
          frame "---------- Process ----------" {
            # "Template Separator\n(You can make a copy of, or modify, this frame)"
            n86 = call <vilib>:"Add State(s) to Queue__jki_lib_state_machine.vi"("State(s) in (\"\")"=w260) -> ("States Out"=w259:string)  [unwired: 14 in]
          }
          frame "Process: Sync" {
            n87 = Unbundle By Name(w268) -> ("Self Reference"=w264:refnum<class "system.lvclass">)
            n88 = call <vilib>:"WaitOnProcessSync.vi"("error in (no error)"=w263, "SMO"=w264) -> ("error out"=w262:errorcluster, "Don't run?"=w267:bool)  [unwired: 7 in, 1 out]
            n89 = Select(t="Data: Cleanup\nEvents: Unregister\nExit", s=w267, f="") -> (s? t:f=w261:string)
            n90 = call <vilib>:"Add State(s) to Queue__jki_lib_state_machine.vi"("State(s) in Front (\"\")"=w261, "State(s) in (\"\")"=w271) -> ("States Out"=w270:string)  [unwired: 13 in]
          }
          frame "---------- Events ----------" {
            # "Template Separator\n(You can make a copy of, or modify, this frame)"
            n91 = call <vilib>:"Add State(s) to Queue__jki_lib_state_machine.vi"("State(s) in (\"\")"=w276) -> ("States Out"=w275:string)  [unwired: 14 in]
          }
          frame "Events: Register" {
            n92 = Unbundle By Name(w293) -> ("Self Reference"=w292:refnum<class "system.lvclass">, "DAQ_Manager"=w291:refnum<class "DAQ_Manager.lvclass">, "DSP"=w290:refnum<class "DSP.lvclass">, "Generator"=w289:refnum<class "Generator.lvclass">)
            n93 = call "lockin.GetEvents.RenameMe.vi"("error in (no error)"=w284, "system in"=w292) -> ("error out"=w279:errorcluster, "System"=w288:T27)  [unwired: 8 in]
            n94 = call "DAQ_Manager.GetEvents.vi"("error in (no error)"=w284, "DAQ_Manager in"=w291) -> ("error out"=w280:errorcluster, "DAQ_Manager"=w281:T30)  [unwired: 8 in]
            n95 = call "DSP.GetEvents.vi"("error in (no error)"=w284, "DSP in"=w290) -> ("error out"=w282:errorcluster, "DSP"=w286:T32)  [unwired: 8 in]
            n96 = call "Generator.GetEvents.vi"("error in (no error)"=w284, "Generator in"=w289) -> ("error out"=w283:errorcluster, "Generator"=w285:T34)  [unwired: 8 in]
            n97 = register-events(w288, w281, w286, w285) -> (reference out=w287:refnum<event-registration>, error out=w277:errorcluster)  [unwired: 2 in]
            n98 = Merge Errors(w277, w279, w280, w282, w283) -> (w278:errorcluster)
            n99 = call <vilib>:"Add State(s) to Queue__jki_lib_state_machine.vi"("State(s) in (\"\")"=w295) -> ("States Out"=w294:string)  [unwired: 14 in]
          }
          frame "Events: Unregister" {
            n100 = Unregister For Events(event registration refnum=w298, error in=w297) -> (error out=w296:errorcluster)
            n101 = call <vilib>:"Clear Errors.vi"("error in (no error)"=w296) -> ()  [unwired: 5 in, 2 out]
            n102 = call <vilib>:"Add State(s) to Queue__jki_lib_state_machine.vi"("State(s) in (\"\")"=w301) -> ("States Out"=w300:string)  [unwired: 14 in]
          }
          frame "---------- system ----------" {
            n103 = call <vilib>:"Add State(s) to Queue__jki_lib_state_machine.vi"("State(s) in (\"\")"=w306) -> ("States Out"=w305:string)  [unwired: 14 in]
          }
          frame "system: template" {
            n104 = Unbundle By Name(w310) -> ("Self Reference"=w308:refnum<class "system.lvclass">)
            n105 = Bundle By Name(cluster=w310, "Self Reference"=w308) -> (w309:T22)
            n106 = call <vilib>:"Add State(s) to Queue__jki_lib_state_machine.vi"("State(s) in (\"\")"=w313) -> ("States Out"=w312:string)  [unwired: 14 in]
          }
          frame "system: DSP" {
            n107 = Unbundle By Name(w321) -> ("Self Reference"=w322:refnum<class "system.lvclass">)
            n108 = Unbundle By Name(w321) -> ("AI Array"=w320:waveform(dbl)[])
            n109 = Unbundle By Name(w322) -> ("DSP"=w316:refnum<class "DSP.lvclass">)
            n110 = call "DSP.setWaveform.vi"("error in (no error)"=w319, "setWaveform"=w320, "DSP"=w316) -> ("error out"=w318:errorcluster, "DSP out"=w315:refnum<class "DSP.lvclass">)  [unwired: 7 in]
            n111 = disable-structure shown="Disabled" {
              disable-tunnel: w318 -> [w329 _]
              disable-tunnel: [w328 _] -> w317
              disable-tunnel: w315 -> [w327 _]
              disable-tunnel: "runCalculation" -> [w326 _]
              frame Disabled {
                n112 = call "DSP.RunCalculation.vi"("error in (no error)"=w329, "runCalculation"=w326, "DSP"=w327) -> ("error out"=w328:errorcluster)  [unwired: 7 in, 1 out]
              }
              frame Enabled {
              }
            }
            n113 = call <vilib>:"Add State(s) to Queue__jki_lib_state_machine.vi"("State(s) in (\"\")"=w325) -> ("States Out"=w324:string)  [unwired: 14 in]
          }
          frame "system: generate" {
            n114 = Unbundle By Name(w331) -> ("Self Reference"=w332:refnum<class "system.lvclass">)
            n115 = Unbundle By Name(w332) -> ()  [unwired: 1 out]
            n116 = call <vilib>:"Add State(s) to Queue__jki_lib_state_machine.vi"("State(s) in (\"\")"=w335) -> ("States Out"=w334:string)  [unwired: 14 in]
          }
          frame "system: write" {
            # "send events out to lockin test launcher"
            n117 = Unbundle By Name(w342) -> ("Self Reference"=w339:refnum<class "system.lvclass">, "AO Array"=w336:waveform(dbl)[])
            n118 = Unbundle By Name(w339) -> ("DAQ_Manager"=w338:refnum<class "DAQ_Manager.lvclass">)
            n119 = call "DAQ_Manager.setWaveforms.vi"("error in (no error)"=w337, "setWaveforms"=w336, "DAQ_Manager"=w338) -> ("error out"=w340:errorcluster)  [unwired: 7 in, 1 out]
            n120 = call "lockin.write.vi"("error in (no error)"=w340, "Write"=w336, "lockin"=w339) -> ("error out"=w341:errorcluster)  [unwired: 7 in, 1 out]
            n121 = call <vilib>:"Add State(s) to Queue__jki_lib_state_machine.vi"("State(s) in (\"\")"=w345) -> ("States Out"=w344:string)  [unwired: 14 in]
          }
        }
      }
    }
    frame Error {
    }
  }
  n122 = call-parent "Process.vi"("error in"=w7, "instrument"=w6) -> ("error out"=w4:errorcluster, "instrument out"=→"system out":refnum<class "system.lvclass">)  [unwired: 8 in]
  n123 = Merge Errors(w4, w3) -> (→"error out":errorcluster)
